vi "generateUUIDs.vi"(6 "timeout (10000)":i32=10000, 8 "error in (no error)":errorcluster, 11 "Parameters":T2) -> (0 "error out":errorcluster, 3 "Response":T1, 4 "error data":string[](array[string]))   [LabVIEW 2017, in "Random JSON API.lvlib"]
uses:
  Random JSON API.lvlib
  Type Defs/generateUUIDsRequest.ctl
  Type Defs/generateUUIDsResponse.ctl
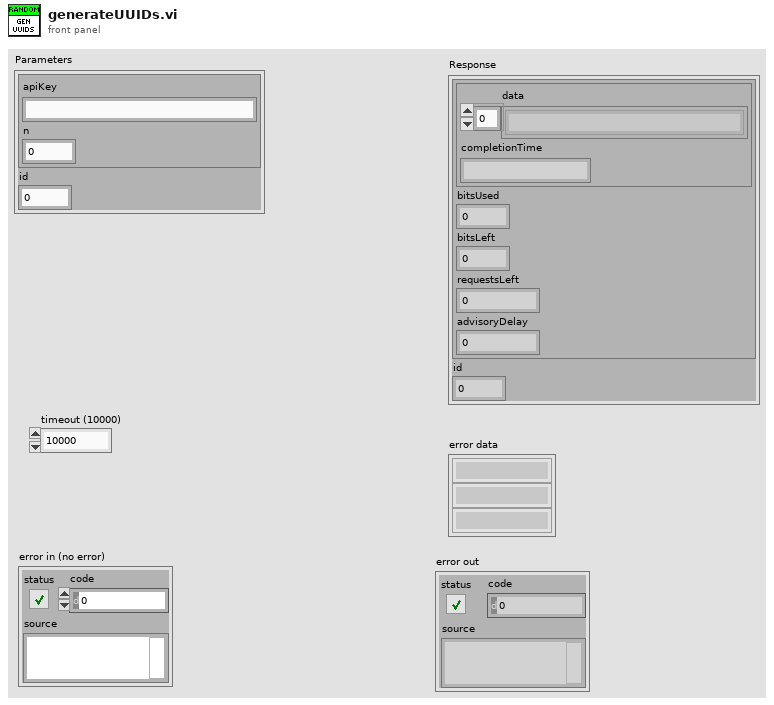
[diagram p1: front panel]
types:
  T1 = typedef "Random JSON API.lvlib/generateUUIDsResponse.ctl" = cluster{"result":cluster{"random":cluster{"data":string[], "completionTime":string}, "bitsUsed":i32, "bitsLeft":i32, "requestsLeft":i32, "advisoryDelay":i32}, "id":dbl}
  T2 = typedef "Random JSON API.lvlib/generateUUIDsRequest.ctl" = cluster{"params":cluster{"apiKey":string, "n":i32}, "id":dbl}
  T3 = cluster{"jsonrpc":string, "method":string, "params":cluster{"apiKey":string, "n":i32}, "id":dbl}
  T4 = cluster{"completionTime":string, "bitsUsed":i32, "bitsLeft":i32, "requestsLeft":i32, "advisoryDelay":i32}
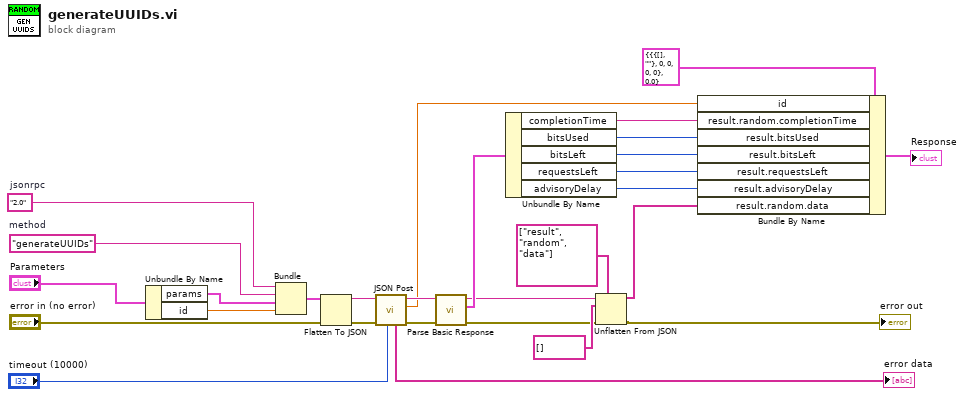
[diagram p0: block diagram]
diagram:
  w18 = "2.0"  # jsonrpc
  w17 = "generateUUIDs"  # method
  n1 = Unbundle By Name("Parameters") -> ("params"=w16:cluster{"apiKey":string, "n":i32}, "id"=w15:dbl)
  n2 = Bundle("jsonrpc"=w18, "method"=w17, "params"=w16, "id"=w15) -> (w14:T3)  [unwired: 1 in]
  n3 = Flatten To JSON(anything=w14, error in (no error)="error in (no error)") -> (JSON string=w21:string, 11:w20:errorcluster)  [unwired: 1 in]
  n4 = call "JSON Post.vi"("timeout (10000)"="timeout (10000)", "error in (no error)"=w20, "Request JSON String"=w21) -> ("error out"=w27:errorcluster, "id"=w8:dbl, "Response JSON String"=w9:string, "error data"=→"error data":string[])  [unwired: 5 in]
  n5 = call "Parse Basic Response.vi"("error in (no error)"=w27, "body in"=w9) -> ("error out"=w4:errorcluster, "result cluster"=w10:T4, "body out"=w7:string)  [unwired: 7 in]
  n6 = Unbundle By Name(w10) -> ("completionTime"=w26:string, "bitsUsed"=w25:i32, "bitsLeft"=w24:i32, "requestsLeft"=w23:i32, "advisoryDelay"=w22:i32)
  n7 = Unflatten From JSON(path=string[] ["result", "random", "data"], JSON string=w7, type and defaults=string[] [], error in (no error)=w4) -> (value=w6:string[], error out=→"error out":errorcluster)  [unwired: 3 in]
  n8 = Bundle By Name(cluster=T1 {"result"={"random"={"data"=[], "completionTime"=""}, "bitsUsed"=0, "bitsLeft"=0, "requestsLeft"=0, "advisoryDelay"=0}, "id"=0.0} ("Response"), "id"=w8, "result.random.completionTime"=w26, "result.bitsUsed"=w25, "result.bitsLeft"=w24, "result.requestsLeft"=w23, "result.advisoryDelay"=w22, "result.random.data"=w6) -> (→"Response":T1)
